vi "Flock_Shared_Destroy Queues.vi"(8 "error in (no error)":errorcluster) -> (0 "error out":errorcluster)   [LabVIEW 2013, in "Flock_Shared_Messaging.lvlib" / "Flock_Shared_CentralProcessMessaging.lvlib"]
uses:
  Flock_Shared_CentralProcessMessaging.lvlib
  Flock_Shared_Messaging.lvlib
  FGV_Action.ctl
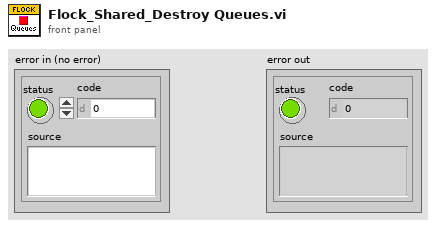
[diagram p1: front panel]
types:
  T1 = typedef "FGV_Action.ctl" = enum16{"Initalize Central", "Initialize Local", "Get", "Delete Local"}
  T2 = typedef "amc_Message Queue.ctl" = refnum<queue>
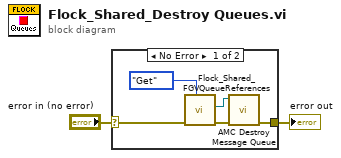
[diagram p0: block diagram]
diagram:
  n1 = case shown="No Error" "error in (no error)" {
    selector: "error in (no error)" -> [w4 w8]
    tunnel: [w3 w8] -> w1
    frame No Error {
      n2 = call "Flock_Shared_FGVQueueReferences.vi"("Action"=FGV_Action."Get", "error in (no error)"=w4) -> ("error out"=w5:errorcluster, "Central Queue out"=w6:T2)  [unwired: 7 in, 1 out]
      n3 = call <vilib>:"AMC Destroy Message Queue.vi"("error in (no error)"=w5, "Message Queue in"=w6) -> ("error out"=w3:errorcluster)  [unwired: 8 in, 1 out]
    }
    frame Error {
    }
  }
  "error out" <- w1
